vi "NetCDFTest.vi"() -> ()   [LabVIEW 2012]
uses:
  <vilib>/Platform/storage/lvStorage.llb/_openFunction.ctl
  <vilib>/Platform/storage/Storage.llb/usiSequenceRepresentation.ctl
  <vilib>/Platform/storage/Storage.llb/usiOverwriteOptions.ctl
  <vilib>/Platform/storage/lvStorage.llb/_defaultFilePath.vi
  <vilib>/Platform/storage/lvStorage.llb/_openStorageWithRootAutoDetect.vi
  <vilib>/Platform/storage/lvStorage.llb/xStorage/xStorageSupp/ErrorOut.vi
  <vilib>/Platform/storage/Storage.llb/_createExplicitChildObject.vi
  <vilib>/Platform/storage/lvStorage.llb/_prepDDT.vi
  <vilib>/Platform/storage/lvStorage.llb/_getChannelNameFromDDT.vi
  <vilib>/Platform/storage/lvStorage.llb/_saveDDT.vi
  <vilib>/Platform/storage/Storage.llb/Get Object Info.vi
  <vilib>/Platform/storage/Storage.llb/__closeStorageFromObject.vi
  <vilib>/Platform/storage/lvStorage.llb/xStorage/Open Data Storage/Open Data Storage.xnode
  <vilib>/Platform/storage/lvStorage.llb/xStorage/Write Data/Write Data.xnode
  <vilib>/Platform/storage/lvStorage.llb/xStorage/Close Data Storage/Close Data Storage.xnode
  <vilib>/measure/NI_MABase.lvlib
panel:
  in  "Path Input":path=path "C:/Users/eol-lidar-admin/Desktop/test.nc"
  out "Path Output":path
  out "error out":errorcluster
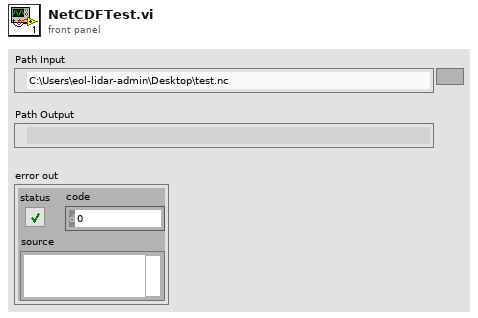
[diagram p1: front panel]
types:
  T1 = enum16{"open", "open or create", "create or replace", "create", "open (read only)"}
  T2 = enum16{"Append values", "Replace values at index", "Replace all values"}
  T3 = enum16{"UPDATE", "READ", "QUERY", "CREATE CHILD", "CREATE", "CONNECT", "DISCONNECT"}
  T4 = typedef "usiOverwriteOptions.ctl" = enum16{"Append values", "Replace values at index", "Replace all values", "Append if timeline aligns"}
  T5 = typedef "usiSequenceRepresentation.ctl" = enum16{"explicit", "implicit"}
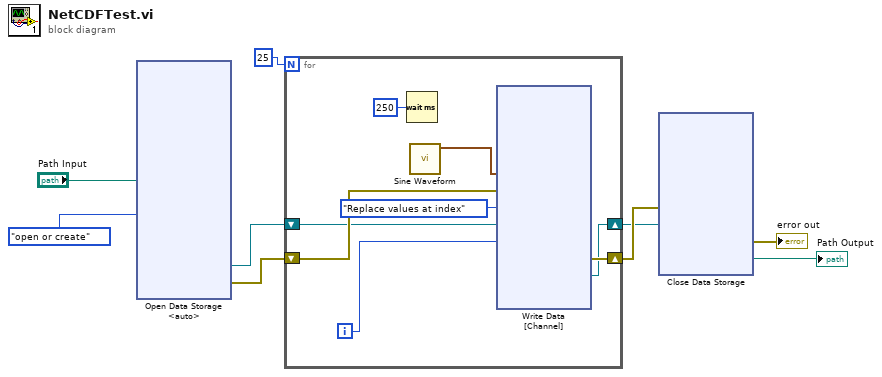
[diagram p0: block diagram]
diagram:
  n1 = xnode "Open Data Storage\n<auto>"("file path"="Path Input", "function (open:0)"=T1."open or create") -> ("storage refnum (file)"=w3:refnum<k20>, "error out"=w4:errorcluster)  [unwired: 3 in, 1 out]
  n2 = for {
    N: 25 -> [_]
    shift-right: [w17] -> w8
    shift-left: w4 -> [w16]
    shift-right: [w15] -> w7
    shift-left: w3 -> [w14]
    i -> [w11]
    n3 = Wait (ms)(milliseconds to wait=u32 250) -> ()  [unwired: 1 out]
    n4 = call <vilib>:"Sine Waveform.vi"() -> ("signal out"=w10:waveform(dbl))  [unwired: 10 in, 1 out]
    n5 = xnode "Write Data\n[Channel]"("Signal"=w10, "error in"=w16, "append / replace (append data values)"=T2."Replace values at index", "storage refnum (file)"=w14, "index"=w11) -> ("error out"=w17:errorcluster, "storage refnum (file) out"=w15:refnum<k20>)  [unwired: 1 out]
  }
  n6 = xnode "Close Data Storage\n"("error in (no error)"=w8, "storage refnum (file)"=w7) -> ("error out"=→"error out":errorcluster, "file path"=→"Path Output":path)
